vi "subDAQ_SetDigStates.vi"(8 "Error in (no error)":errorcluster, 10 "Digital line array":tag[](array[tag])=["Dev1/port0/line0"], 11 "Digital States (Value) array":bool[](array[boolean])) -> (0 "Error out":errorcluster)   [LabVIEW 2015]
uses:
  <vilib>/DAQmx/write.llb/DAQmx Write (Digital 1D Bool NChan 1Samp 1Line).vi
  <vilib>/DAQmx/create/channels.llb/DAQmx Create Channel (DO-Digital Output).vi
  <vilib>/DAQmx/miscellaneous.llb/DAQmx Fill In Error Info.vi
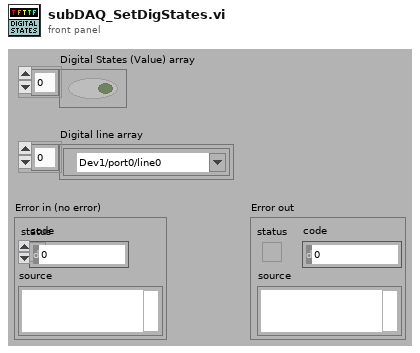
[diagram p1: front panel]
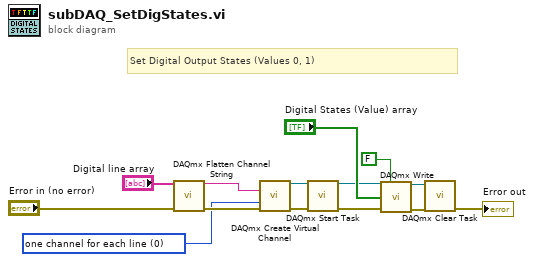
[diagram p0: block diagram]
diagram:
  w8 = 0 items=["one channel for each line", "one channel for all lines"] ("line grouping")
  # "Set Digital Output States (Values 0, 1)"
  n1 = call <vilib>:"DAQmx Flatten Channel String.vi"("names in"="Digital line array", "error in"="Error in (no error)") -> ("names out"=w7:string, "error out"=w14:errorcluster)  [unwired: 12 out]
  n2 = call-poly <vilib>:"DAQmx Create Virtual Channel.vi"("lines"=w7, "line grouping"=w8, "error in"=w14) -> ("task out"=w10:refnum<k21>, "error out"=w9:errorcluster)  [unwired: 2 in, 9 out]
  n3 = call <vilib>:"DAQmx Start Task.vi"("task/channels in"=w10, "error in"=w9) -> ("task out"=w6:refnum<k21>, "error out"=w5:errorcluster)  [unwired: 12 out]
  n4 = call-poly <vilib>:"DAQmx Write.vi"("task/channels in"=w6, "auto start"=FALSE, "data"="Digital States (Value) array", "error in"=w5) -> ("task out"=w3:refnum<k21>, "error out"=w2:errorcluster)  [unwired: 10 out]
  n5 = call <vilib>:"DAQmx Clear Task.vi"("task in"=w3, "error in"=w2) -> ("error out"=→"Error out":errorcluster)  [unwired: 13 out]
